vi "Disabled.vi"(7 "Robot Mode":T2, 10 "Match Info":T1={"Autonomous Elapsed Seconds"=0.0, "TeleOp Elapsed Seconds"=0.0, "Disabled Elapsed Seconds"=0.0, "Visited Autonomous"=FALSE, "Visited TeleOp"=FALSE, "Visited Disabled"=FALSE, "Autonomous Settings"={"Autonomous Style"=enum."Independent", "VI Refnum"=refnum}}, 11 "Call Context":T3) -> ()   [LabVIEW 2014]
doc: "This VI is called each time a disabled packet is received from the DS. It is often used to prepare for the next robot mode, to calibrate sensors, etc."
uses:
  <vilib>/Rock Robotics/WPI/DriverStation/WPI_DriverStationDerivedRobotMode.ctl
  <vilib>/Rock Robotics/WPI/DriverStation/WPI_DriverStationRobotMode2.ctl
  <vilib>/Rock Robotics/WPI/DriverStation/WPI_DriverStationMatch Info.ctl
  Drivetrain Code/Drivetrain Control.ctl
  Drivetrain Code/Drivetrain Mode.ctl
  Common Code/Change Detect Boolean.vi
  <vilib>/Rock Robotics/WPI/Joystick/WPI_JoystickGetSetRefNum.vi
  Robot Global Data.vi
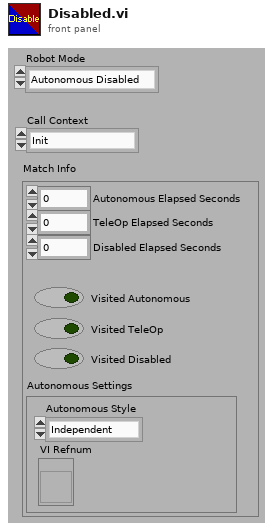
[diagram p1: front panel]
types:
  T1 = typedef "WPI_DriverStationMatch Info.ctl" = cluster{"Autonomous Elapsed Seconds":dbl, "TeleOp Elapsed Seconds":dbl, "Disabled Elapsed Seconds":dbl, "Visited Autonomous":bool, "Visited TeleOp":bool, "Visited Disabled":bool, "Autonomous Settings":cluster{"Autonomous Style":enum16{"Iterative", "Independent"}, "VI Refnum":refnum<vi>}}
  T2 = typedef "WPI_DriverStationRobotMode2.ctl" = enum16{"Autonomous Disabled", "Autonomous Enabled", "Teleop Disabled", "Teleop Enabled", "Disconnected", "Finish", "Test Disabled", "Test Enabled", "Emergency Stopped"}
  T3 = typedef "WPI_DriverStationDerivedRobotMode.ctl" = enum16{"Init", "Execute", "Stop"}
  T4 = typedef "Drivetrain Control.ctl" = cluster{"Mode":T5, "X":dbl, "Y":dbl, "Heading Target":dbl, "Drive X":dbl, "Drive Y":dbl}
  T5 = typedef "Drivetrain Mode.ctl" = enum16{"Manual", "Gyro Steer", "Vision Steer", "Drive Distance"}
  T6 = typedef "WPI_JoystickDevRef.ctl" = cluster{"Device":T7}
  T7 = typedef "WPI_JoystickDeviceEnum.ctl" = enum16{"USB 0", "USB 1", "USB 2", "USB 3", "USB 4", "USB 5"}
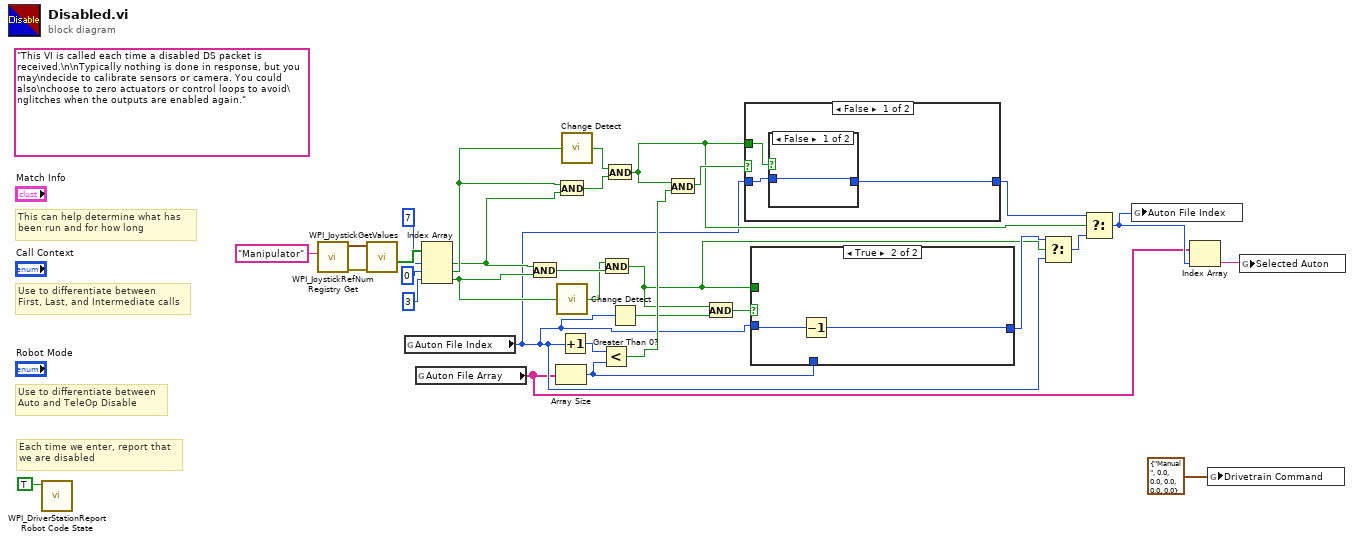
[diagram p0: block diagram]
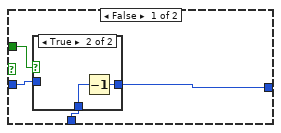
[diagram p2: hidden frame]
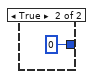
[diagram p4: hidden frame]
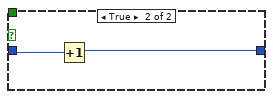
[diagram p5: hidden frame]
diagram:
  (unwired) "This VI is called each time a disabled DS packet is received.\n\nTypically nothing is done in response, but you may\ndecide to calibrate sensors or camera. You could also\nchoose to zero actuators or control loops to avoid\nglitches when the outputs are enabled again."
  # "Each time we enter, report that\nwe are disabled"
  # "Use to differentiate between\nFirst, Last, and Intermediate calls"
  # "This can help determine what has\nbeen run and for how long"
  # "Use to differentiate between\nAuto and TeleOp Disable"
  n1 = call <vilib>:"WPI_DriverStationReport Robot Code State.vi"("Disabled"=TRUE ("Autonomous")) -> ()  [unwired: 10 in, 1 out]
  n2 = call <vilib>:"WPI_JoystickRefNum Registry Get.vi"("refnum name"="Manipulator") -> ("error out"=w30:errorcluster, "JoystickDevRef"=w29:T6)  [unwired: 9 in]
  n3 = call <vilib>:"WPI_JoystickGetValues.vi"("error in (no error)"=w30, "JoystickDevRef"=w29) -> ("Buttons"=w27:bool[])  [unwired: 5 in, 4 out]
  n4 = global read "Robot Global Data.vi" "Auton File Index"() -> (w4:i32)
  n5 = global read "Robot Global Data.vi" "Auton File Array"() -> (w2:string[])
  n6 = Index Array(array=w27, index #1=7 ("index"), index #2=0 ("index"), index #3=3 ("index")) -> (element #1=w18:bool, element #2=w20:bool, element #3=w19:bool)
  n7 = And(x=w18, y=w19) -> (x .and. y?=w25:bool)
  n8 = Array Size(array=w2) -> (size(s)=w17:i32)
  n9 = And(x=w20, y=w18) -> (x .and. y?=w24:bool)
  n10 = call-poly "Change Detect.vi"("In"=w19) -> ("Changed?"=w5:bool)
  n11 = Increment(x=w4) -> (x+1=w23:i32)
  n12 = call-poly "Change Detect.vi"("In"=w20) -> ("Changed?"=w6:bool)
  n13 = Less?(x=w23, y=w17) -> (x < y?=w16:bool)
  n14 = And(x=w5, y=w25) -> (x .and. y?=w9:bool)
  n15 = And(x=w6, y=w24) -> (x .and. y?=w10:bool)
  n16 = Greater Than 0?(x=w4) -> (x > 0?=w7:bool)
  n17 = And(x=w10, y=w16) -> (x .and. y?=w15:bool)
  n18 = And(x=w9, y=w7) -> (x .and. y?=w12:bool)
  n19 = case shown="False" w15 {
    tunnel: w4 -> [w34 w38]
    tunnel: w10 -> [w33 _]
    tunnel: [w32 w37] -> w14
    frame False {
      n20 = case shown="False" w33 {
        tunnel: [w35 0 ("Auton File Index")] -> w32
        tunnel: w34 -> [w35 _]
        frame False {
        }
        frame True {
        }
      }
    }
    frame True {
      n21 = Increment(x=w38) -> (x+1=w37:i32)
    }
  }
  n22 = case shown="True" w12 {
    tunnel: w4 -> [w42 w47]
    tunnel: w9 -> [w41 _]
    tunnel: w17 -> [w40 _]
    tunnel: [w39 w46] -> w11
    frame False {
      n23 = case shown="True" w41 {
        tunnel: [w43 w45] -> w39
        tunnel: w42 -> [w43 _]
        tunnel: w40 -> [_ w44]
        frame False {
        }
        frame True {
          n24 = Decrement(x=w44) -> (x-1=w45:i32)
        }
      }
    }
    frame True {
      n25 = Decrement(x=w47) -> (x-1=w46:i32)
    }
  }
  n26 = Select(t=w11, s=w9, f=w4) -> (s? t:f=w13:i32)
  n27 = Select(t=w14, s=w10, f=w13) -> (s? t:f=w8:i32)
  n28 = global write "Robot Global Data.vi" "Auton File Index"(w8) -> ()
  n29 = Index Array(array=w2, index=w8) -> (element=w3:string)
  n30 = global write "Robot Global Data.vi" "Drivetrain Command"(T4 {"Mode"=enum."Manual", "X"=0.0, "Y"=0.0, "Heading Target"=0.0, "Drive X"=0.0, "Drive Y"=0.0} ("Drivetrain Command")) -> ()
  n31 = global write "Robot Global Data.vi" "Selected Auton"(w3) -> ()
